vi "LinkDeviceReadWrite.vi"() -> (2 "Table Control":string[][](table))   [LabVIEW 2024]
uses:
  C:/Users/chrismadlax/Desktop/LabVIEW-BLE-Driver/BLELib.dll
  BLELib.dll
panel:
  in  "LinkDevice":bool
  in  "RAWAddress":u64=69987970987151
  in  "CharacteristicUUID":string="19b10001-e8f2-537e-4f6c-d104768a1214"
  out "Numeric":i32
  out "Result":string
  in  "Boolean":bool
  out "ServicesUUIDs Value":string
  out "Pair Result":string
  # "Arduino BLE 33 board RAWaddress"
  # "A4:DA:32:0D:F5:E2"
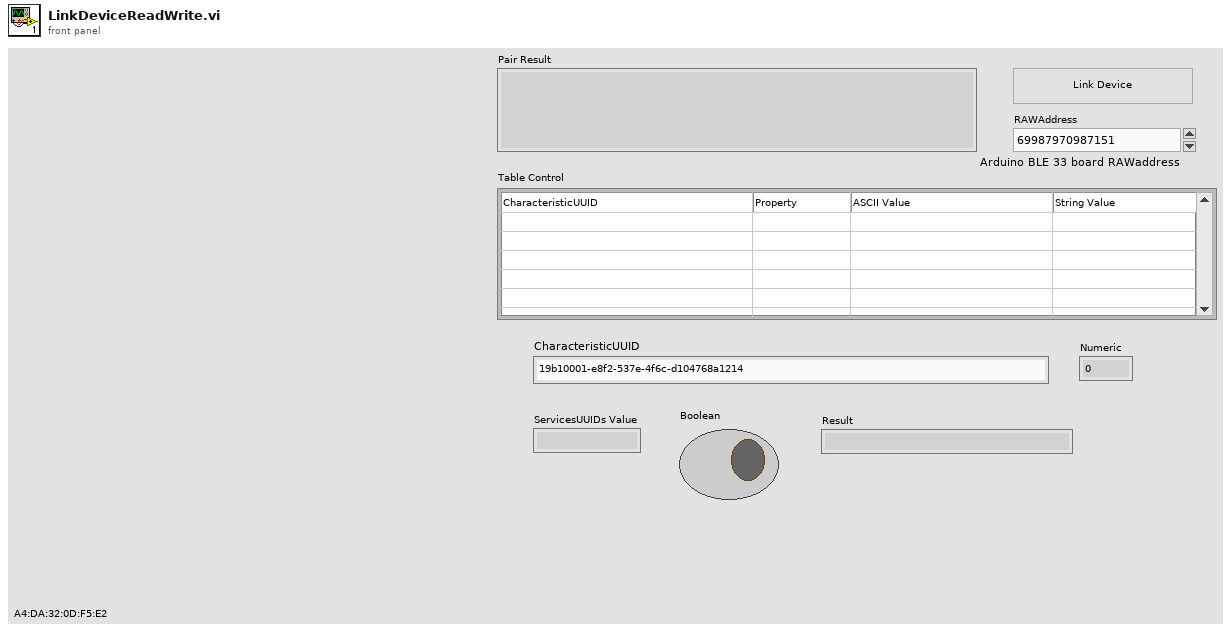
[diagram p1: front panel]
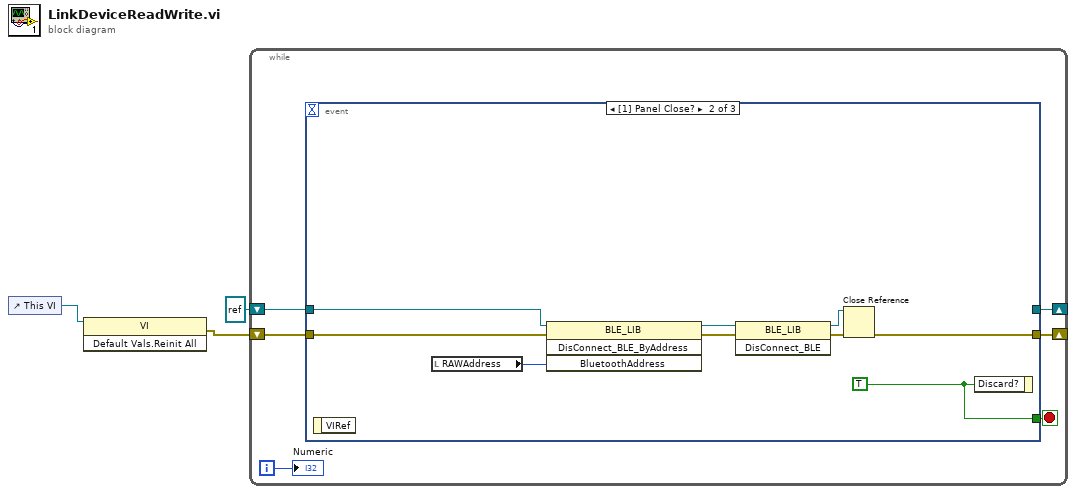
[diagram p0: block diagram]
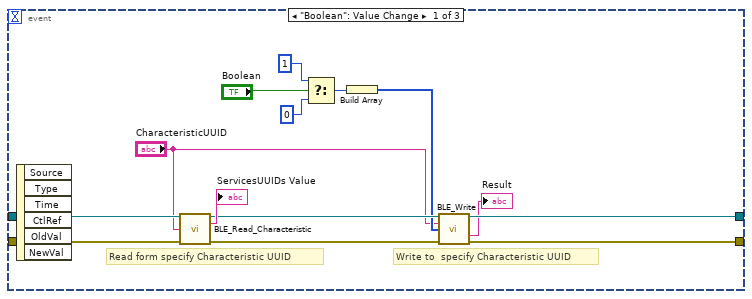
[diagram p2: hidden frame]
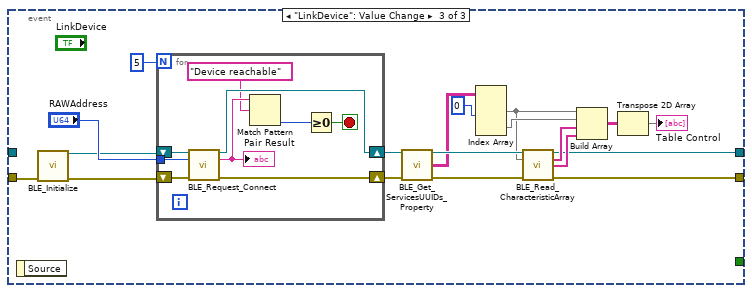
[diagram p3: hidden frame]
diagram:
  n1 = control-ref of="This VI"() -> (w1:refnum<vi>)
  n2 = invoke class="VI" method="Default Vals.Reinit All"(reference=w1) -> (error out=w2:errorcluster)  [unwired: 2 in, 2 out]
  n3 = while {
    shift-right: [w6] -> _
    shift-left: refnum<k24> refnum (".NET Refnum out") -> [w9]
    shift-right: [w7] -> _
    shift-left: w2 -> [w8]
    i -> [w5]
    stop <- w4 stop-if-true
    n4 = event shown="[1] Panel Close?" {
      selector: _ -> [_ _ _]
      dyn-events: _ -> [_ _ _]
      timeout: _ -> [_ _ _]
      tunnel: w9 -> [w23 w25 _]
      tunnel: w8 -> [w22 w27 w35]
      tunnel: [w19 w26 w37] -> w7
      tunnel: [w17 _ w36] -> w6
      tunnel: [_ w32 _] -> w4
      event "Boolean": Value Change {
        # "Write to  specify Characteristic UUID"
        # "Read form specify Characteristic UUID"
        n5 = event-data() -> ()  [unwired: 1 in, 6 out]
        n6 = call "BLE_Read_Characteristic.vi"(".NET Refnum in"=w23, "CharacteristicUUID"="CharacteristicUUID", "error in (no error)"=w22) -> (".NET Refnum out"=w18:refnum<k24>, "ServicesUUIDs Value"=→"ServicesUUIDs Value":string, "error out"=w21:errorcluster)  [unwired: 8 in, 2 out]
        n7 = Select(t=u8 1, s="Boolean", f=u8 0) -> (s? t:f=w14:u8)
        n8 = Build Array(w14) -> (w11:u8[])
        n9 = call "BLE_Write.vi"(".NET Refnum in"=w18, "UUID"="CharacteristicUUID", "WriteByteArray"=w11, "error in (no error)"=w21) -> (".NET Refnum out"=w17:refnum<k24>, "Result"=→"Result":string, "error out"=w19:errorcluster)  [unwired: 9 in]
      }
      event Panel Close? {
        w32 = TRUE ("Discard?")
        n10 = event-data() -> ()  [unwired: 1 in, 1 out]
        n11 = local read "RAWAddress"() -> (w24:u64)
        n12 = invoke class="BLE_LIB" method="DisConnect_BLE_ByAddress"(reference=w25, error in=w27, "BluetoothAddress"=w24) -> (reference out=w31:refnum<k24>, error out=w29:errorcluster)  [unwired: 1 in, 2 out]
        n13 = invoke class="BLE_LIB" method="DisConnect_BLE"(reference=w31, error in=w29) -> (reference out=w30:refnum<k24>, error out=w28:errorcluster)  [unwired: 1 in, 1 out]
        n14 = Close Reference(reference=w30, error in (no error)=w28) -> (error out=w26:errorcluster)
        n15 = event-data("Discard?"=w32) -> ()  [unwired: 1 in, 1 out]
      }
      event "LinkDevice": Value Change {
        n16 = event-data() -> ()  [unwired: 1 in, 1 out]
        n17 = call "BLE_Initialize.vi"("error in (no error)"=w35) -> (".NET Refnum out"=w34:refnum<k24>, "error out"=w33:errorcluster)  [unwired: 13 in]
        n18 = for {
          N: 5 -> [_]
          tunnel: "RAWAddress" -> [w58]
          shift-right: [w56] -> w41
          shift-left: w33 -> [w60]
          shift-right: [w57] -> w40
          shift-left: w34 -> [w59]
          stop <- w52 stop-if-true
          n19 = call "BLE_Request_Connect.vi"(".NET Refnum in"=w59, "BluetoothAddress"=w58, "error in (no error)"=w60) -> (".NET Refnum out"=w57:refnum<k24>, "ConnectBLE"=w55:string, "error out"=w56:errorcluster)  [unwired: 10 in]
          "Pair Result" <- w55
          n20 = Match Pattern(string=w55, regular expression="Device reachable") -> (offset past match=w53:i32)  [unwired: 1 in, 3 out]
          n21 = Greater Or Equal To 0?(x=w53) -> (x >= 0?=w52:bool)
        }
        n22 = call "BLE_Get_ServicesUUIDs_Property.vi"(".NET Refnum in"=w40, "error in (no error)"=w41) -> (".NET Refnum out"=w50:refnum<k24>, "Char Val-Property"=w48:string[][], "error out"=w49:errorcluster)  [unwired: 11 in]
        n23 = Index Array(array=w48, index (col) #1=0 ("disabled index (col)")) -> (element #1=w45:string[], element #2=w46:string[])  [unwired: 3 in]
        n24 = call "BLE_Read_CharacteristicArray.vi"(".NET Refnum in"=w50, "ServicesUUIDs Extract Value"=w45, "error in (no error)"=w49) -> (".NET Refnum out"=w36:refnum<k24>, "ServicesUUIDs ASCII Value"=w42:string[], "ServicesUUIDs Value"=w43:string[], "error out"=w37:errorcluster)  [unwired: 9 in]
        n25 = Build Array(w45, w46, w42, w43) -> (w44:string[][])
        n26 = Transpose 2D Array(2D array=w44) -> (transposed array=→"Table Control":string[][])
      }
    }
    "Numeric" <- w5
  }
